vi "RX.vi"(8 "error in (no error)":errorcluster, 9 "RX":bool, 10 "Data":u8[](array[numeric]), 11 "Vision in":refnum<class "Vision.lvclass">) -> (0 "error out":errorcluster, 3 "Vision out":refnum<class "Vision.lvclass">)   [LabVIEW 2022 SP3, in "Vision.lvlib" / "Vision.lvclass"]
uses:
  Vision.lvclass
  Vision.lvclass/Vision.ctl
  Phoenix/Phoenix Messages/Vision RX Msg/Vision RX Msg.lvclass
  <vilib>/ActorFramework/Actor/Actor.lvclass
  C:/Program Files (x86)/National Instruments/LabVIEW 2022/vi.lib/ActorFramework/Actor/Actor.lvclass
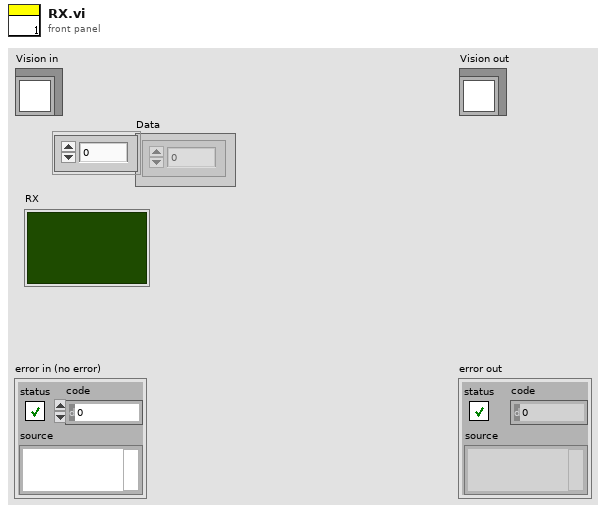
[diagram p1: front panel]
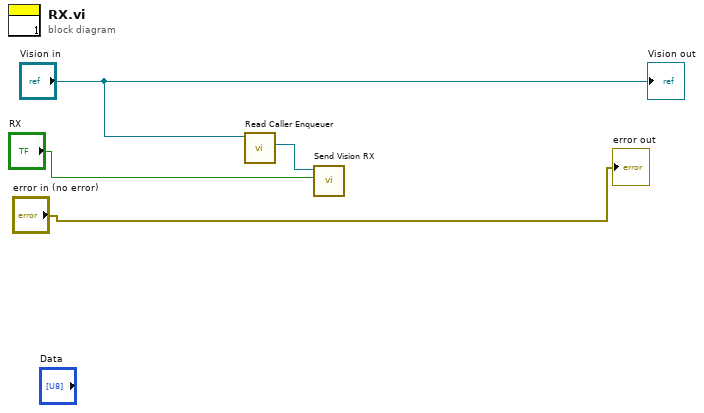
[diagram p0: block diagram]
diagram:
  n1 = call <vilib>:"Read Caller Enqueuer.vi"("Actor"="Vision in") -> ("Caller Enqueuer"=w1:refnum<class "Message Enqueuer.lvclass">)  [unwired: 10 in]
  n2 = call "Send Vision RX.vi"("RX"="RX", "Message Enqueuer"=w1) -> ()  [unwired: 8 in, 2 out]
  "error out" <- "error in (no error)"
  "Vision out" <- "Vision in"
